vi "Process data.vi"(6 "Numeric":u32, 7 "data":dbl[][](array[numeric]), 9 "Array 5":dbl[](array[numeric]), 10 "Array 4":dbl[](array[numeric]), 11 "Array 8":dbl[](array[numeric])) -> (0 "Array 7":dbl[](array[numeric]), 1 "Array":dbl[][](array[numeric]), 2 "Array 9":dbl[](array[numeric]), 3 "Array 2":dbl[](array[numeric]), 4 "Array 3":dbl[][](array[numeric]), 5 "Array 6":dbl[](array[numeric]))   [LabVIEW 2018]
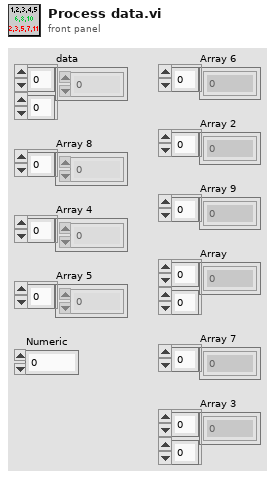
[diagram p1: front panel]
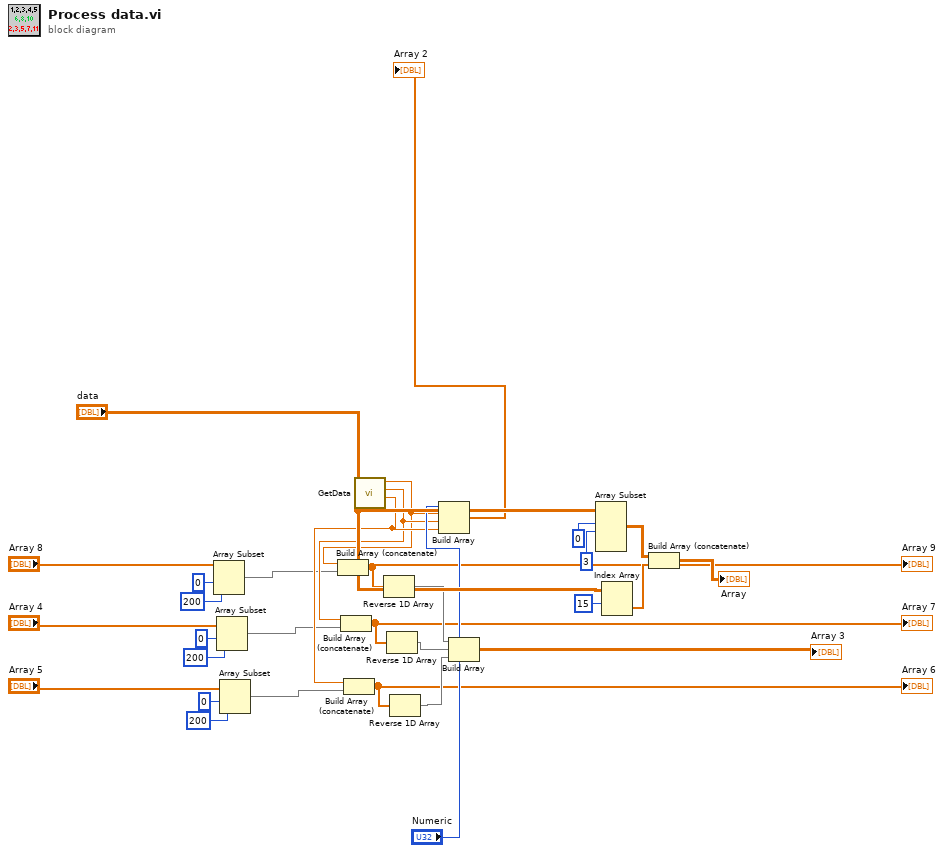
[diagram p0: block diagram]
diagram:
  n1 = Array Subset(array="Array 8", index=0, length=200) -> (w3:dbl[])
  n2 = Array Subset(array="Array 4", index=0, length=200) -> (w8:dbl[])
  n3 = Array Subset(array="Array 5", index=0, length=200) -> (w11:dbl[])
  n4 = call "GetData.vi"("data"="data") -> ("mean 405"=w21:dbl, "mean 470"=w20:dbl, "F470-F405/F405"=w19:dbl)  [unwired: 8 in]
  n5 = Build Array (concatenate)(w19, w3) -> (w4:dbl[])
  "Array 9" <- w4
  n6 = Build Array (concatenate)(w20, w8) -> (w12:dbl[])
  "Array 7" <- w12
  n7 = Build Array (concatenate)(w21, w11) -> (w13:dbl[])
  "Array 6" <- w13
  n8 = Reverse 1D Array(array=w4) -> (reversed array=w17:dbl[])
  n9 = Reverse 1D Array(array=w12) -> (reversed array=w16:dbl[])
  n10 = Reverse 1D Array(array=w13) -> (reversed array=w18:dbl[])
  n11 = Build Array("Numeric", w19, w20, w21) -> (→"Array 2":dbl[])
  n12 = Build Array(w17, w16, w18) -> (→"Array 3":dbl[][])
  n13 = Array Subset(array="data", index (row)=0, length (row)=3 ("length")) -> (w28:dbl[][])  [unwired: 2 in]
  n14 = Index Array(array="data", index (row)=15) -> (element=w29:dbl[])  [unwired: 1 in]
  n15 = Build Array (concatenate)(w28, w29) -> (→"Array":dbl[][])
